vi "PathPlanner_CommandUtil_TrajIssue.vi"(11 "Command":T1) -> ()   [LabVIEW 2019, in "PathPlanner24.lvlib"]
doc: "Issues the given command.\n\nCurrently the only type of commands that can be issued are Boolean commands. The value is forced to TRUE when the command is issued.\n\nThe following table lists the actions performed for different types of commands:\n - Unknown - nothing - not supported.\n - Wait - nothing - not supported\n - Named - Issue boolean command with TRUE value using the \"name\" as the command name.\n - Path - nothing - not supported\n - Sequential, Parallel, Race, Deadline - Issue boolean command with TRUE value for each of the commands contained in the \"commands\" array. The value for \"name\" is used as the command name.\n\nInputs:\n -- Command - cluster - Command definition.\n\nOutputs:\n -- <none>"
uses:
  PathPlanner24.lvlib
  ENum/PathPlanner_CommandUtil_Type_ENUM.ctl
  TypeDef/PathPlannerCommandUtil.ctl
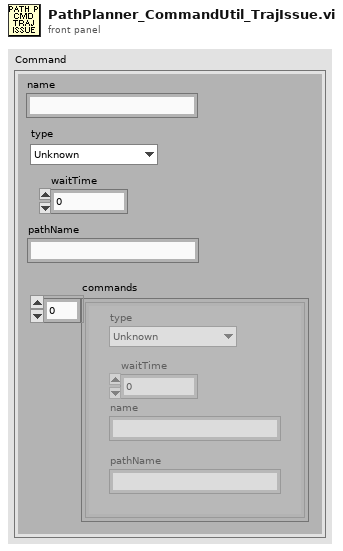
[diagram p1: front panel]
types:
  T1 = typedef "PathPlanner24.lvlib/PathPlannerCommandUtil.ctl" = cluster{"waitTime":dbl, "name":string, "pathName":string, "commands":cluster{"type":T2, "waitTime":dbl, "name":string, "pathName":string}[], "type":T2}
  T2 = typedef "PathPlanner24.lvlib/PathPlanner_CommandUtil_Type_ENUM.ctl" = enum16{"Unknown", "Wait", "Named", "Path", "Sequential", "Parallel", "Race", "Deadline", "PointTowardsZoneEnter", "PointTowardsZoneExit", "TriggerEventStart", "TriggerEventStop", "TriggerEventOneshot"}
  T3 = cluster{"type":T2, "waitTime":dbl, "name":string, "pathName":string}[]
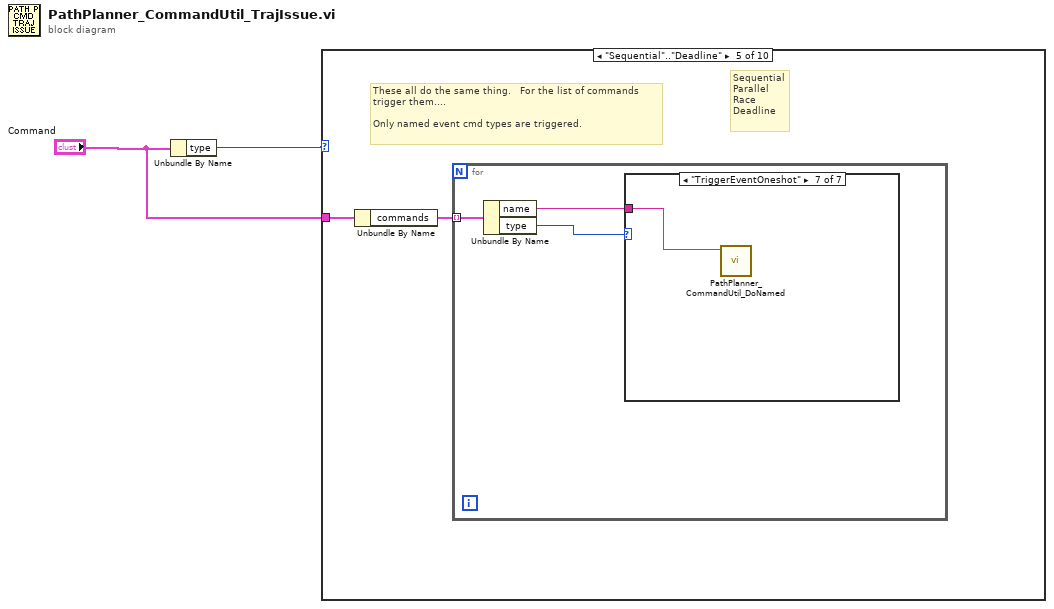
[diagram p0: block diagram]
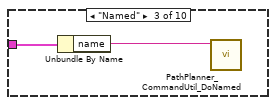
[diagram p4: hidden frame]
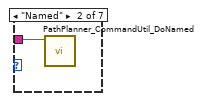
[diagram p7: hidden frame]
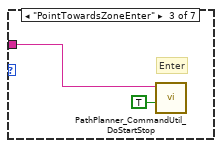
[diagram p8: hidden frame]
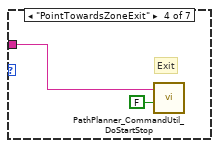
[diagram p9: hidden frame]
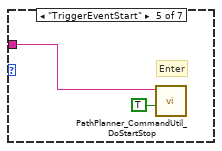
[diagram p10: hidden frame]
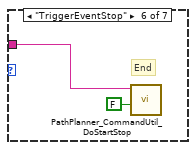
[diagram p11: hidden frame]
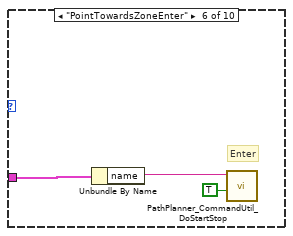
[diagram p12: hidden frame]
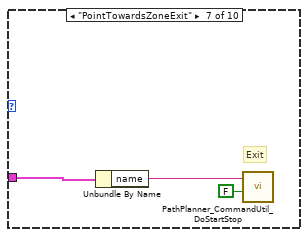
[diagram p13: hidden frame]
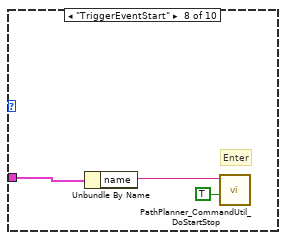
[diagram p14: hidden frame]
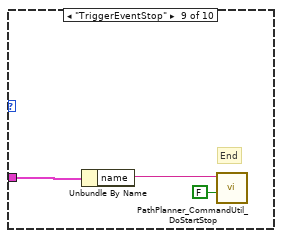
[diagram p15: hidden frame]
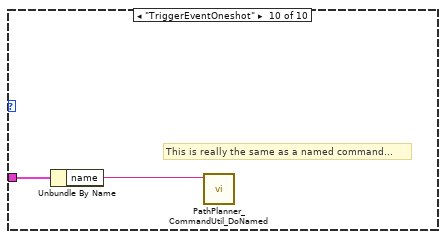
[diagram p16: hidden frame]
diagram:
  n1 = Unbundle By Name("Command") -> ("type"=w2:T2)
  n2 = case shown="\"Sequential\"..\"Deadline\"" w2 {
    tunnel: "Command" -> [_ _ w4 _ w6 w22 w25 w26 w29 w32]
    frame "Unknown" {
      # "Unknown -- do nothiing"
    }
    frame "Wait" {
      # "Cant just stop while running a trajectory...."
      # "Wait - do nothing..."
    }
    frame "Named" {
      n3 = Unbundle By Name(w4) -> ("name"=w3:string)
      n4 = call "PathPlanner_CommandUtil_DoNamed.vi"("Event Action Name"=w3) -> ()  [unwired: 11 in]
    }
    frame "Path" {
      # "Already running a trajectory.... Should this stop and run a new one???"
      # "Do nothing.....  for now..."
    }
    frame "Sequential".."Deadline" {
      # "Sequential\nParallel\nRace\nDeadline"
      # "These all do the same thing.   For the list of commands\ntrigger them....\n\nOnly named event cmd types are triggered."
      n5 = Unbundle By Name(w6) -> ("commands"=w5:T3)
      n6 = for {
        tunnel: w5 -> [w9] mode=indexing
        n7 = Unbundle By Name(w9) -> ("name"=w8:string, "type"=w7:T2)
        n8 = case shown="\"TriggerEventOneshot\"" w7 {
          tunnel: w8 -> [_ w10 w11 w13 w15 w17 w19]
          frame "Unknown", Default {
          }
          frame "Named" {
            n9 = call "PathPlanner_CommandUtil_DoNamed.vi"("Event Action Name"=w10) -> ()  [unwired: 11 in]
          }
          frame "PointTowardsZoneEnter" {
            # "Enter"
            n10 = call "PathPlanner_CommandUtil_DoStartStop.vi"("Enter_Exit"=TRUE, "Event Action Name"=w11) -> ()  [unwired: 10 in]
          }
          frame "PointTowardsZoneExit" {
            # "Exit"
            n11 = call "PathPlanner_CommandUtil_DoStartStop.vi"("Enter_Exit"=FALSE, "Event Action Name"=w13) -> ()  [unwired: 10 in]
          }
          frame "TriggerEventStart" {
            # "Enter"
            n12 = call "PathPlanner_CommandUtil_DoStartStop.vi"("Enter_Exit"=TRUE, "Event Action Name"=w15) -> ()  [unwired: 10 in]
          }
          frame "TriggerEventStop" {
            # "End"
            n13 = call "PathPlanner_CommandUtil_DoStartStop.vi"("Enter_Exit"=FALSE, "Event Action Name"=w17) -> ()  [unwired: 10 in]
          }
          frame "TriggerEventOneshot" {
            n14 = call "PathPlanner_CommandUtil_DoNamed.vi"("Event Action Name"=w19) -> ()  [unwired: 11 in]
          }
        }
      }
    }
    frame "PointTowardsZoneEnter" {
      # "Enter"
      n15 = Unbundle By Name(w22) -> ("name"=w20:string)
      n16 = call "PathPlanner_CommandUtil_DoStartStop.vi"("Enter_Exit"=TRUE, "Event Action Name"=w20) -> ()  [unwired: 10 in]
    }
    frame "PointTowardsZoneExit" {
      # "Exit"
      n17 = Unbundle By Name(w25) -> ("name"=w24:string)
      n18 = call "PathPlanner_CommandUtil_DoStartStop.vi"("Enter_Exit"=FALSE, "Event Action Name"=w24) -> ()  [unwired: 10 in]
    }
    frame "TriggerEventStart" {
      # "Enter"
      n19 = Unbundle By Name(w26) -> ("name"=w27:string)
      n20 = call "PathPlanner_CommandUtil_DoStartStop.vi"("Enter_Exit"=TRUE, "Event Action Name"=w27) -> ()  [unwired: 10 in]
    }
    frame "TriggerEventStop" {
      # "End"
      n21 = Unbundle By Name(w29) -> ("name"=w30:string)
      n22 = call "PathPlanner_CommandUtil_DoStartStop.vi"("Enter_Exit"=FALSE, "Event Action Name"=w30) -> ()  [unwired: 10 in]
    }
    frame "TriggerEventOneshot" {
      # "This is really the same as a named command..."
      n23 = Unbundle By Name(w32) -> ("name"=w33:string)
      n24 = call "PathPlanner_CommandUtil_DoNamed.vi"("Event Action Name"=w33) -> ()  [unwired: 11 in]
    }
  }
